vi "Scale Data.vi"(9 "Data":dbl[][](array[numeric]), 11 "DataProcessor in":refnum<class "DataProcessor.lvclass">) -> (1 "Scaled Data":dbl[][](array[numeric]), 3 "DataProcessor out":refnum<class "DataProcessor.lvclass">)   [LabVIEW 2020, in "Volatus.lvlib" / "DataProcessor.lvclass"]
uses:
  DataProcessor.lvclass
  DataProcessor.lvclass/DataProcessor.ctl
  Polynomial Remove Trailing Zeros.vi
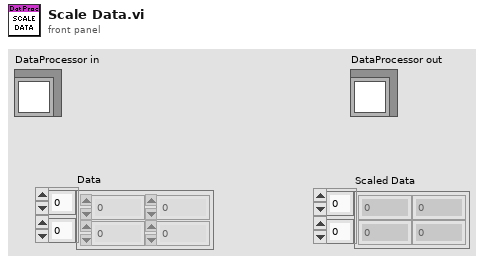
[diagram p1: front panel]
types:
  T1 = typedef "VolatusConfig.lvlib/Scale Type.ctl" = enum16{"None", "Sensor", "Polynomial", "Threshold"}
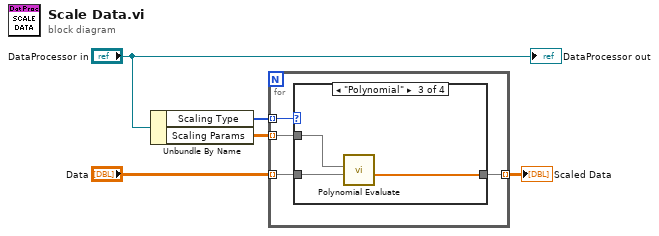
[diagram p0: block diagram]
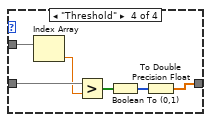
[diagram p4: hidden frame]
diagram:
  n1 = Unbundle By Name("DataProcessor in") -> ("Scaling Type"=w1:T1[], "Scaling Params"=w2:dbl[][])
  n2 = for {
    tunnel: w2 -> [w9] mode=indexing
    tunnel: "Data" -> [w8] mode=indexing
    tunnel: [w7] -> w4 mode=indexing
    tunnel: w1 -> [w6] mode=indexing
    n3 = case shown="\"Polynomial\"" w6 {
      tunnel: w9 -> [_ _ w14 w20]
      tunnel: w8 -> [w10 w11 w13 w19]
      tunnel: [w10 w11 w12 w16] -> w7
      frame "None" {
      }
      frame "Sensor" {
        # "#ERROR?\nSensor should be converted to another type."
      }
      frame "Polynomial" {
        n4 = call "Polynomial Evaluate.vi"("Data"=w13, "Coefficients"=w14) -> ("Results"=w12:dbl[])  [unwired: 9 in]
      }
      frame "Threshold" {
        n5 = Index Array(array=w20) -> (element=w18:dbl)  [unwired: 1 in]
        n6 = Greater?(x=w19, y=w18) -> (0:w15:bool[])
        n7 = Boolean To (0,1)(Boolean=w15) -> (0, 1=w17:i16[])
        n8 = To Double Precision Float(number=w17) -> (double precision float=w16:dbl[])
      }
    }
  }
  "Scaled Data" <- w4
  "DataProcessor out" <- "DataProcessor in"
